vi "tunnel M2-M2.5.vi"(5 "I2C Ref in":T1, 8 "error in (no error)":errorcluster) -> (0 "error out":errorcluster, 2 "I2C Ref Out":T1)   [LabVIEW 2017]
uses:
  <vilib>/myRIO/Instrument Drivers/Onboard IO/I2C/typedefs/I2C Reference.ctl
  <vilib>/myRIO/Common/Instrument Driver Framework/Utilities/typedefs/myRIO Generic Hardware Reference.ctl
  <vilib>/myRIO/Common/Instrument Driver Framework/Utilities/typedefs/Hardware Version Enum.ctl
  <vilib>/myRIO/Common/Instrument Driver Framework/Utilities/typedefs/myRIO v1.0 Reference.ctl
  <vilib>/myRIO/Common/Instrument Driver Framework/Utilities/typedefs/Generic FPGA Reference.ctl
  <vilib>/myRIO/Common/Instrument Driver Framework/myRIO v1.0/I2C/typedefs/I2C Channels Enum.ctl
  <vilib>/myRIO/Instrument Drivers/Onboard IO/I2C/typedefs/I2C Configuration.ctl
  <vilib>/myRIO/Instrument Drivers/Onboard IO/I2C/typedefs/I2C Transfer Rate.ctl
  <vilib>/myRIO/Instrument Drivers/Onboard IO/I2C/I2C.lvlib
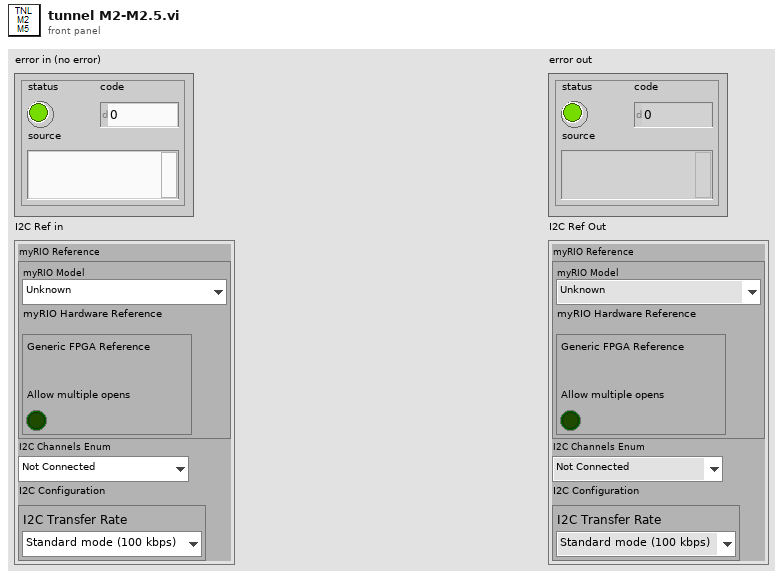
[diagram p1: front panel]
types:
  T1 = typedef "I2C.lvlib/I2C Reference.ctl" = cluster{"myRIO Reference":T2, "I2C Channels Enum":T6, "I2C Configuration":T7}
  T2 = typedef "myRIO Generic Hardware Reference.ctl" = cluster{"myRIO Model":T3, "myRIO Hardware Reference":T4}
  T3 = typedef "Hardware Version Enum.ctl" = enum16{"Unknown", "myRIO-1900", "myRIO-1950", "roboRIO", "NI ELVIS RIO CM"}
  T4 = typedef "myRIO v1.0 Reference.ctl" = cluster{"Generic FPGA Reference":T5, "Allow multiple opens":bool}
  T5 = typedef "Generic FPGA Reference.ctl" = refnum<k20>
  T6 = typedef "I2C Channels Enum.ctl" = enum16{"Not Connected", "A/I2C", "B/I2C", "I2C/I2C"}
  T7 = typedef "I2C.lvlib/I2C Configuration.ctl" = cluster{"I2C Transfer Rate":T8}
  T8 = typedef "I2C.lvlib/I2C Transfer Rate.ctl" = enum16{"Standard mode (100 kbps)", "Fast mode (400 kbps)"}
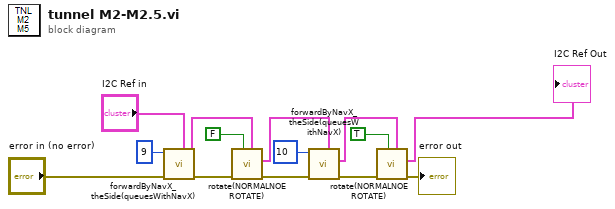
[diagram p0: block diagram]
diagram:
  n1 = call "forwardByNavX_theSide(queuesWithNavX).vi"("I2C Ref Out"="I2C Ref in", "error in (no error)"="error in (no error)", "distance the side"=u32 9) -> ("error out"=w12:errorcluster, "I2C Ref Out 2"=w4:T1)  [unwired: 7 in]
  n2 = call "rotate(NORMALNOE ROTATE).vi"("I2C Ref in"=w4, "On/Off\nRight/Left"=FALSE ("On/Off\nRight/Left"), "error in (no error)"=w12) -> ("error out"=w11:errorcluster, "I2C Ref out"=w3:T1)  [unwired: 7 in]
  n3 = call "forwardByNavX_theSide(queuesWithNavX).vi"("I2C Ref Out"=w3, "error in (no error)"=w11, "distance the side"=u32 10) -> ("error out"=w10:errorcluster, "I2C Ref Out 2"=w2:T1)  [unwired: 7 in]
  n4 = call "rotate(NORMALNOE ROTATE).vi"("I2C Ref in"=w2, "On/Off\nRight/Left"=TRUE ("On/Off\nRight/Left"), "error in (no error)"=w10) -> ("error out"=→"error out":errorcluster, "I2C Ref out"=→"I2C Ref Out":T1)  [unwired: 7 in]
